vi "Untitled 2.vi"() -> ()   [LabVIEW 2016]
uses:
  <vilib>/ptbypt/NI_PtbyPt.lvlib
panel:
  out "X Values":dbl[](array[numeric])
  out "x*y":dbl
  in  "Stop":bool
  in  "intervals":i32=10
  in  "Make Measurement":bool=TRUE
  out "Histogram Graph":T1(graph)
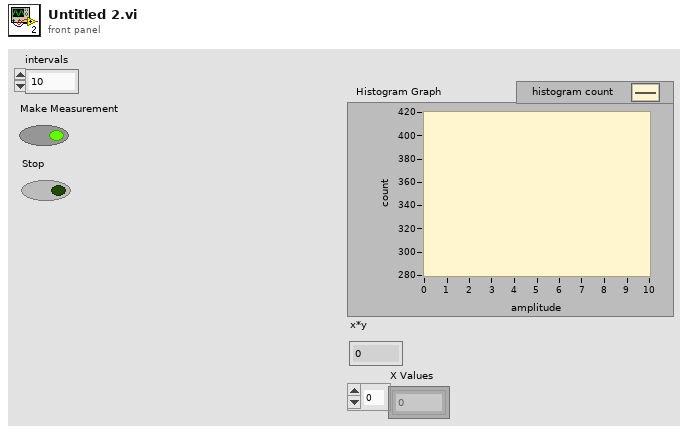
[diagram p1: front panel]
types:
  T1 = cluster{"X Values":dbl[], "Histogram: h(x)":i32[]}
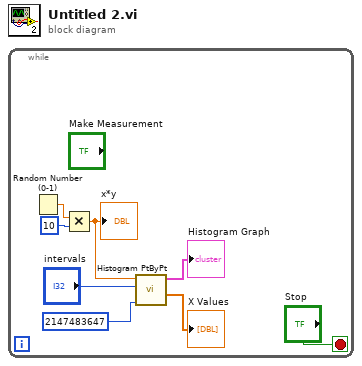
[diagram p0: block diagram]
diagram:
  n1 = while {
    stop <- "Stop" stop-if-true
    n2 = Random Number (0-1)() -> (number: 0 to 1=w6:dbl)
    n3 = Multiply(x=w6, y=10) -> (x*y=w4:dbl)
    "x*y" <- w4
    n4 = call <vilib>:"Histogram PtByPt.vi"("sample length"=2147483647, "intervals"="intervals", "x"=w4) -> ("X Values"=→"X Values":dbl[], "Histogram Graph"=→"Histogram Graph":T1)  [unwired: 5 in, 2 out]
  }
